vi "getAngle.vi"(6 "Channel":i32, 8 "error in (no error)":errorcluster, 11 "Instrument.Cryostat in":refnum<class "Instrument.Cryostat.lvclass">) -> (0 "error out":errorcluster, 1 "Status":string, 2 "Angle (°)":dbl, 3 "Instrument.Cryostat out":refnum<class "Instrument.Cryostat.lvclass">, 4 "Finished?":bool)   [LabVIEW 2019, in "Instrument.Cryostat.lvclass"]
uses:
  Instrument.Cryostat.lvclass
  Typedefs/getAngle--cluster.ctl
  Typedefs/Cryostat.commands--enum.ctl
  273053de-a208-493c-8017-50a26cb4e47e.vi
  273053de-a208-493c-8017-50a26cb4e47e.vi/15d12a34-2780-498e-ac80-39b3f44422b0.vi
  273053de-a208-493c-8017-50a26cb4e47e.vi/0107df6e-2d6b-482e-9ca6-de5f7e2cb1e1.vi
  <vilib>/Utility/Data Type/Get Type Information.vi
  <vilib>/JDP Science/JSONtext/JSON text to Variant.vi
  <vilib>/JDP Science/JSONtext/LVClass Serializer/JSONtext LVClass Serializer.lvclass
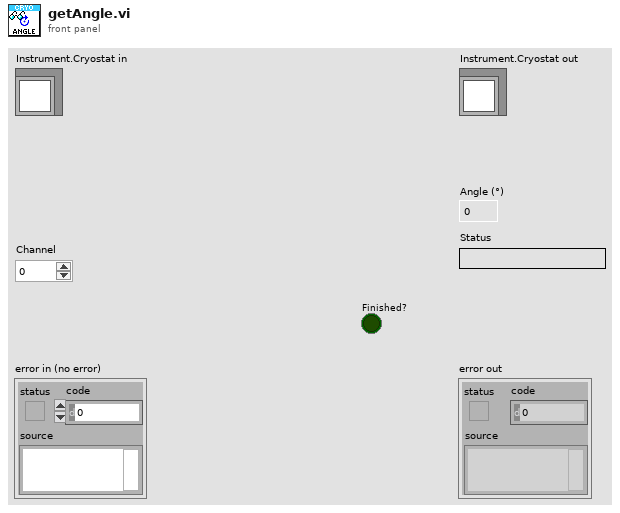
[diagram p1: front panel]
types:
  T1 = typedef "Instrument.Cryostat.lvclass/Cryostat.commands--enum.ctl" = enum16{"getLN2Level", "getLHeLevel", "getMagnet", "getMagnetVector", "setMagnet", "setMagnetVector", "getAngle", "setAngle", "getTemperature", "setTemperature", "getHeater", "setHeater", "getChamber", "setChamber", "getPressure"}
  T2 = typedef "Instrument.Cryostat.lvclass/getAngle--cluster.ctl" = cluster{"angle":dbl, "status":string, "finished":bool}
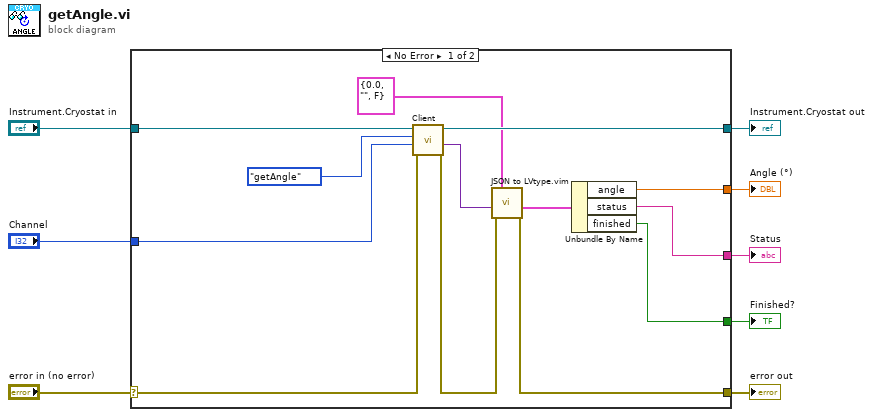
[diagram p0: block diagram]
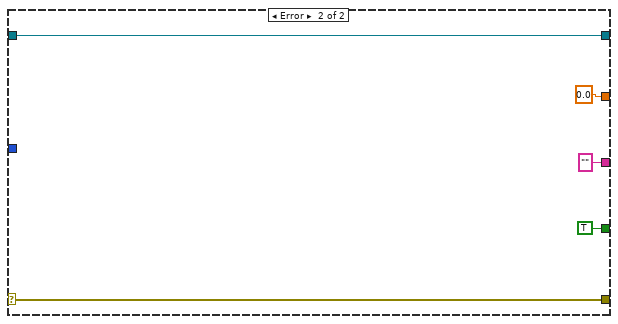
[diagram p2: hidden frame]
diagram:
  n1 = case shown="No Error" "error in (no error)" {
    selector: "error in (no error)" -> [w15 w26]
    tunnel: [w9 w26] -> w7
    tunnel: [w21 w25] -> w5
    tunnel: "Instrument.Cryostat in" -> [w16 w25]
    tunnel: "Channel" -> [w20 _]
    tunnel: [w19 0.0 ("Angle (°)")] -> w3
    tunnel: [w18 "" ("Status")] -> w2
    tunnel: [w17 TRUE ("Finished?")] -> w1
    frame No Error {
      n2 = call-dynamic "Client.vi"("error in (no error)"=w15, "Data in"=w20, "Command in"=Cryostat.commands--enum."getAngle" ("commands"), "Instrument in"=w16) -> ("error out"=w10:errorcluster, "Data out"=w13:variant, "Instrument out"=w21:refnum<class "Instrument.Cryostat.lvclass">)  [unwired: 4 in, 1 out]
      n3 = call "JSON to LVtype.vim"("type"=T2 {"angle"=0.0, "status"="", "finished"=FALSE} ("getAngle"), "error in (no error)"=w10, "JSON Data in"=w13) -> ("error out"=w9:errorcluster, "Data out"=w11:T2)  [unwired: 7 in]
      n4 = Unbundle By Name(w11) -> ("angle"=w19:dbl, "status"=w18:string, "finished"=w17:bool)
    }
    frame Error {
    }
  }
  "error out" <- w7
  "Instrument.Cryostat out" <- w5
  "Angle (°)" <- w3
  "Status" <- w2
  "Finished?" <- w1
